vi "24 OS Commands.vi"() -> ()   [LabVIEW 2019]
uses:
  _Subs/OpenDiagram/Open_XControl.xctl
panel:
  out "standard output":string
  in  "OpenDiag":refnum<vi>(xcontrol)
  # "04 OS Commands\nThis code runs a command (directory listing) in the operating system\n\nInstructions:\n1. Hit the Run arrow and see the folders/files\n2. Look at the code - try a different command"
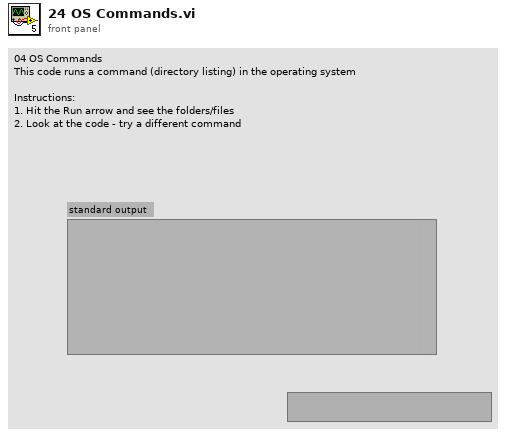
[diagram p1: front panel]
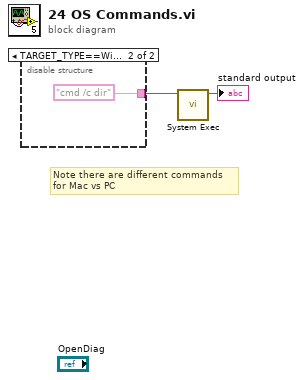
[diagram p0: block diagram]
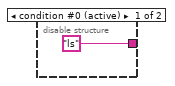
[diagram p2: hidden frame]
diagram:
  # "Note there are different commands\nfor Mac vs PC"
  n1 = disable-structure shown="TARGET_TYPE==Windows" {
    disable-tunnel: ["ls" ("command line") "cmd /c dir" ("command line")] -> w2
    frame condition #0 (active) {
    }
    frame condition #1 {
    }
  }
  n2 = call <vilib>:"System Exec.vi"("command line"=w2) -> ("standard output"=→"standard output":string)  [unwired: 7 in, 3 out]
